vi "bbauv_acoustic_sbRIO_v2.vi"() -> ()   [LabVIEW 2012]
doc: "This VI will initialize the FPGA VI and read a user-defined number of samples from a DMA FIFO. When the data acquisition is complete this VI will read status information from the FPGA VI.\n\nFollow these instructions to run the VI.\n\n1. Select your RIO device from the dropdown.\n2. Set the sample period, number of samples to acquire per channel, and DMA block read size. \n\nNote: the block read size should be set to balance load on the host processor and the update rate of the user interface. A small block read size will update the user interface more often but will result in a higher load on the host processor."
uses:
  <vilib>/userdefined/High Color/nirio_resource_hc.ctl
  <vilib>/Analysis/3filter.llb/Butterworth Filter (DBL).vi
  <vilib>/FPGAPlugInAG/sbRIO-9612/niLvFpga_Open_sbRIO-9612.vi
  <vilib>/rvi/interface/common/dynamic/niFpgaDynamicAddResources.vi
  <vilib>/Utility/error.llb/Error Cluster From Error Code.vi
  <vilib>/FPGAPlugInAG/Dynamic/niLvFpga_Run_Dynamic.vi
  <vilib>/rvi/errors/niLvFpgaAdjustHostInterfaceError.vi
  <vilib>/RVI Host/nirviSupport.llb/nirviErrorClusterFromErrorCode.vi
  <vilib>/FPGAPlugInAG/Dynamic/niLvFpga_Close_Dynamic.vi
  <vilib>/rvi/interface/nirviOpenFPGA/nirviOpenFPGA.xnode
  FPGA Bitfiles/bbauvFPGA_FPGATarget2_NI9223User-Contr_AXBjtBmtN8Y.lvbitx
  NI 9223 User-Controlled IO Sampling (FPGA).vi
  <vilib>/rvi/interface/nirviMethod/nirviMethod.xnode
  <vilib>/rvi/interface/nirviReadWriteControl/nirviReadWriteControl.xnode
  <vilib>/rvi/interface/nirviCloseFPGA/nirviCloseFPGA.xnode
  <vilib>/rvi/errors/niLvFpgaMergeErrorWithErrorCode.vi
  <vilib>/rvi/interface/Simulation/niFpgaSimulationCallBeginRW.vi
  <vilib>/FPGAPlugInAG/Dynamic/niLvFpga_ReadFifo_Dynamic.vi
  <vilib>/rvi/interface/nirviMethod/StockFPGA_InlinedMethodWaitForSingleIRQ.vi
  <vilib>/FPGAPlugInAG/Dynamic/niLvFpga_WaitOnIrq_Dynamic.vi
  <vilib>/FPGAPlugInAG/Dynamic/niLvFpga_AcknowledgeIrq_Dynamic.vi
  NiFpgaLv.dll
  <vilib>/FPGAPlugInAG/Dynamic/niLvFpga_ConfigureFifo_Dynamic.vi
  <vilib>/FPGAPlugInAG/Dynamic/niLvFpga_StartFifo_Dynamic.vi
  <vilib>/Analysis/NI_AALBase.lvlib
  <vilib>/Analysis/NI_AALPro.lvlib
panel:
  in  "threshold ratio":dbl=3.0
  out "Sidemove":dbl
  out "Forward":dbl
  out "Threshold 3":dbl
  out "Threshold 2":dbl
  out "Threshold 1":dbl
  out "noise index":dbl[](array[numeric])
  out "Threshold 0":dbl
  out "Amplitude Spectrum":waveform(dbl)(graph)
  out "bad signal?":bool
  in  "Min Starting Index":i32=7000
  in  "Portion Duration":i32=1000
  out "amplitude 3":dbl
  out "amplitude 2":dbl
  out "amplitude 1":dbl
  out "amplitude 0":dbl
  in  "noise min":dbl=0.001
  out "Index 3":dbl
  out "Index 2":dbl
  out "Index 1":dbl
  out "Index 0":dbl
  out "current time":timestamp
  in  "Debug":bool=TRUE
  in  "Send to ROS":bool
  out "ROS  Error":bool
  out "dt1":dbl
  out "dt2":dbl
  out "dt3":dbl
  out "pitch":dbl
  out "yaw":dbl
  out "z":dbl
  out "y":dbl
  out "x":dbl
  in  "Mode":T1(ring)=enum."Use Far Field"
  in  "Altitude":dbl=2.0
  in  "Display Filtered Signal":bool=TRUE
  out "Ratio at Index (%)":dbl
  out "Selected Index":i32
  in  "Threshold":dbl=0.1
  in  "low cutoff freq: fl":dbl=20000.0
  in  "high cutoff freq: fh":dbl=30000.0
  out "Yaw Chart":dbl(graph)
  out "Ch0 Signal":dbl[](graph)
  out "#Elements Acquired":u32(graph)
  out "Extracted signal":dbl[][](graph)
  in  "Sampling Duration (us)":u32=2005000
  in  "RIO Device":T2="RIO0"
  out "Timed Out":bool
  out "Sample Gated":bool
  out "Overwrite":bool
  in  "Acquisition Stop":bool
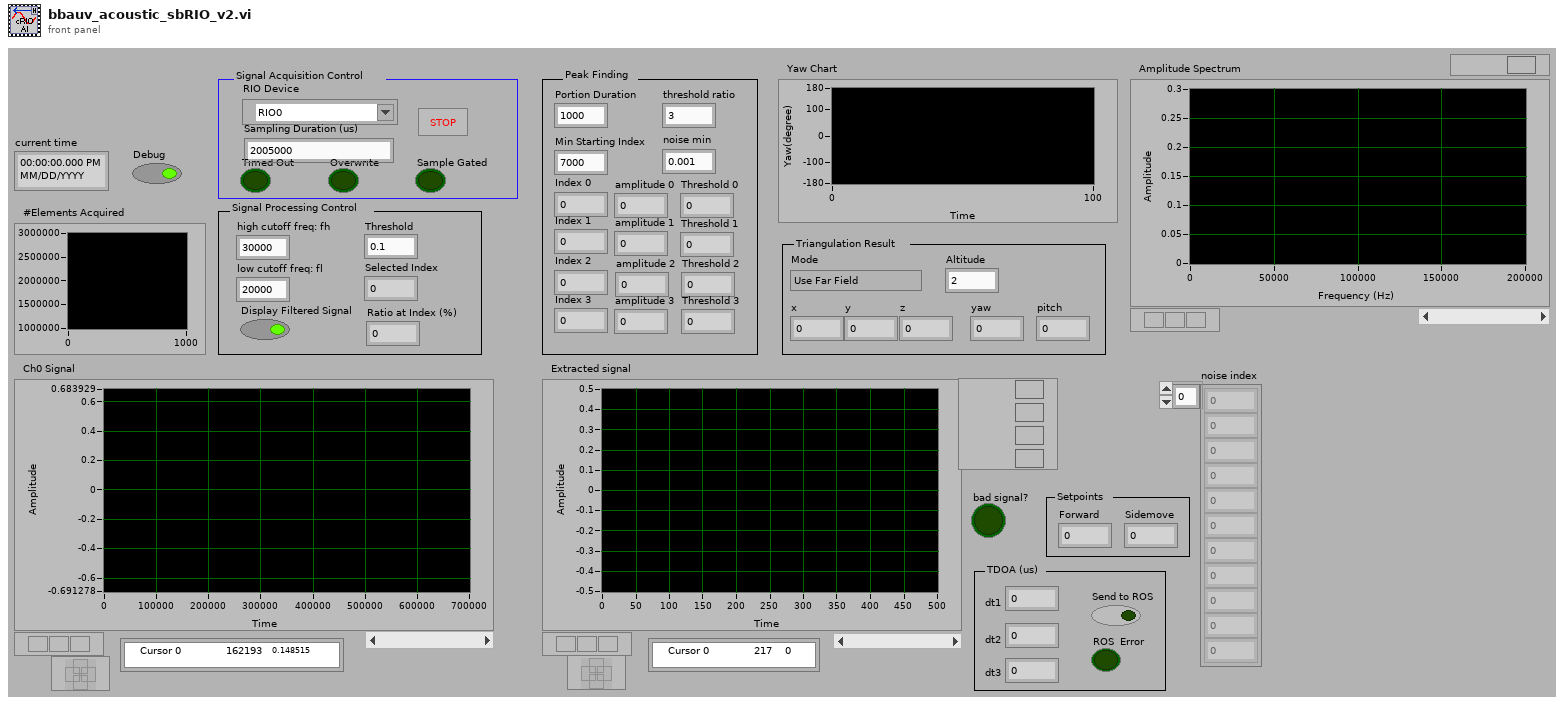
[diagram p1: front panel]
types:
  T1 = enum16{"Use Near Field", "Use Far Field", "Far Field with 3 hydrophones"}
  T2 = typedef "nirio_resource_hc.ctl" = tag
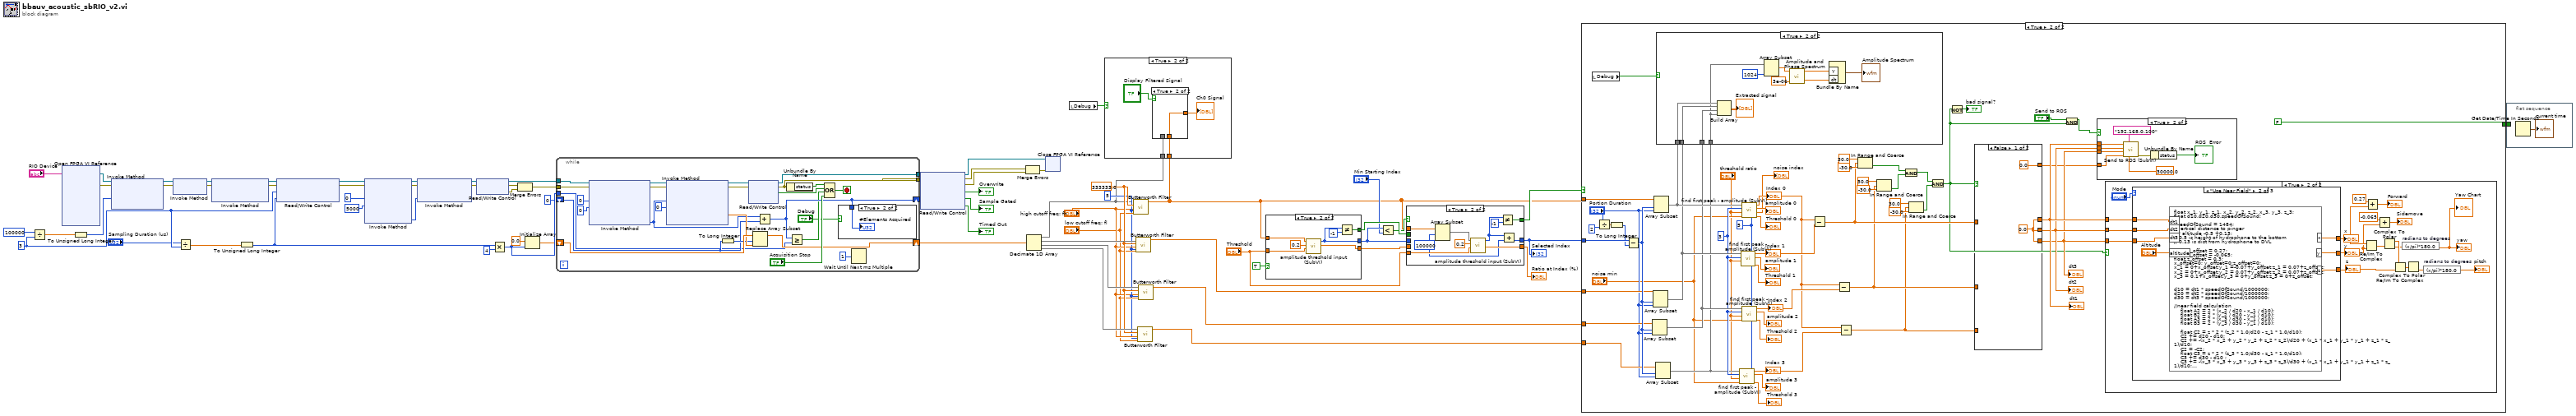
[diagram p0: block diagram]
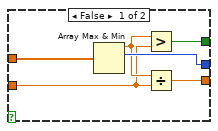
[diagram p5: hidden frame]
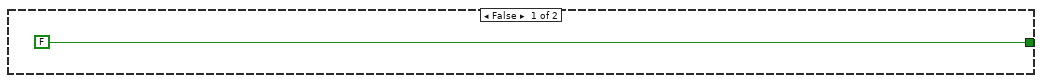
[diagram p6: hidden frame]
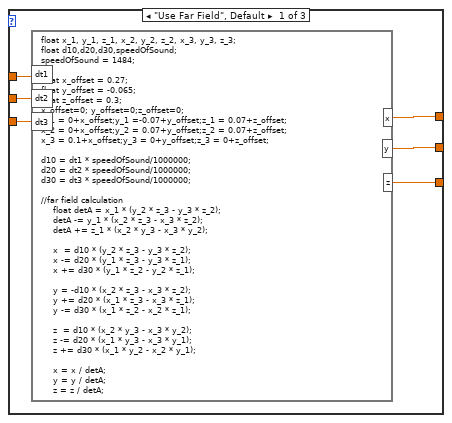
[diagram p8: hidden frame]
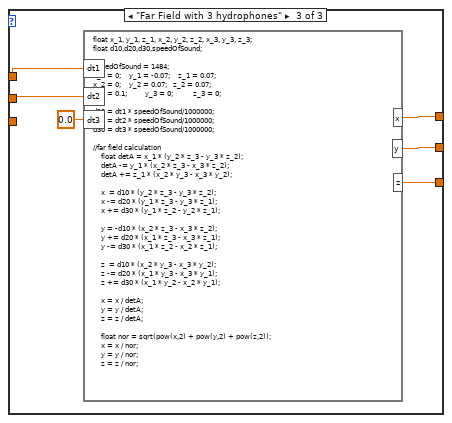
[diagram p9: hidden frame]
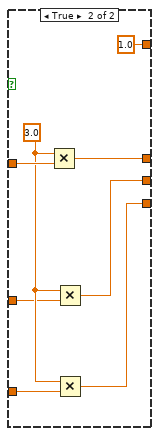
[diagram p11: hidden frame]
diagram:
  w6 = 5
  w12 = 333333.0
  w29 = u32 3
  n1 = Divide(x=u32 100000, y=w29) -> (x/y=w62:dbl)
  n2 = xnode "Open FPGA VI Reference"("resource name"="RIO Device") -> ("FPGA VI Reference Out"=w65:refnum<k20>, "error out"=w64:errorcluster)  [unwired: 1 in]
  n3 = To Unsigned Long Integer(number=w62) -> (unsigned 32bit integer=w63:u32)
  n4 = xnode "Invoke Method"("FPGA VI Reference In"=w65, "error in"=w64, "Requested Depth"=w63) -> ("FPGA VI Reference Out"=w67:refnum<k20>, "error out"=w66:errorcluster)  [unwired: 1 out]
  n5 = xnode "Invoke Method"("FPGA VI Reference In"=w67, "error in"=w66) -> ("FPGA VI Reference Out"=w56:refnum<k20>, "error out"=w55:errorcluster)
  n6 = Divide(x="Sampling Duration (us)", y=w29) -> (x/y=w27:dbl)
  n7 = xnode "Invoke Method"("FPGA VI Reference In"=w56, "error in"=w55) -> ("FPGA VI Reference Out"=w32:refnum<k20>, "error out"=w31:errorcluster)  [unwired: 1 in]
  n8 = To Unsigned Long Integer(number=w27) -> (unsigned 32bit integer=w25:u32)
  n9 = xnode "Read/Write Control"("FPGA VI Reference In"=w32, "error in"=w31, "Sample Period (uSec)"=w29, "Number of Samples"=w25) -> ("FPGA VI Reference Out"=w46:refnum<k20>, "error out"=w45:errorcluster)
  n10 = xnode "Invoke Method"("FPGA VI Reference In"=w46, "error in"=w45, "IRQ Number(s)"=0, "Timeout (ms)"=5000) -> ("FPGA VI Reference Out"=w43:refnum<k20>, "error out"=w44:errorcluster, "IRQ(s) Asserted"=w40:i32)  [unwired: 1 out]
  n11 = xnode "Invoke Method"("FPGA VI Reference In"=w43, "error in"=w44, "IRQ Number(s)"=w40) -> ("FPGA VI Reference Out"=w42:refnum<k20>, "error out"=w41:errorcluster)
  n12 = xnode "Read/Write Control"("FPGA VI Reference In"=w42, "error in"=w41) -> ("FPGA VI Reference Out"=w34:refnum<k20>, "error out"=w48:errorcluster, "Error Out"=w47:errorcluster)
  n13 = Multiply(x=w25, y=u32 4) -> (x*y=w59:u32)
  n14 = Merge Errors(w48, w47) -> (w33:errorcluster)
  n15 = Initialize Array(sgl 0.0, w59) -> (w35:sgl[])
  n16 = while {
    tunnel: w34 -> [w81]
    tunnel: w33 -> [w80]
    tunnel: [w89] -> w54
    tunnel: [w88] -> w53
    shift-right: [w71] -> _
    shift-left: u32 0 -> [w82]
    tunnel: w59 -> [w74]
    shift-right: [w84] -> w26
    shift-left: w35 -> [w90]
    stop <- w91 stop-if-true
    n17 = xnode "Invoke Method"("FPGA VI Reference In"=w81, "error in"=w80, "Number of Elements"=u32 0, "Timeout (ms)"=0) -> ("FPGA VI Reference Out"=w79:refnum<k20>, "error out"=w78:errorcluster, "Elements Remaining"=w72:u32)  [unwired: 1 out]
    n18 = xnode "Invoke Method"("FPGA VI Reference In"=w79, "error in"=w78, "Number of Elements"=w72, "Timeout (ms)"=0) -> ("FPGA VI Reference Out"=w94:refnum<k20>, "error out"=w93:errorcluster, "Data"=w85:sgl[])  [unwired: 1 out]
    n19 = To Long Integer(number=w82) -> (32bit integer=w83:i32)
    n20 = xnode "Read/Write Control"("FPGA VI Reference In"=w94, "error in"=w93) -> ("FPGA VI Reference Out"=w89:refnum<k20>, "error out"=w88:errorcluster, "Error"=w73:bool)  [unwired: 1 out]
    n21 = Replace Array Subset(array=w90, new element=w85, index=w83) -> (w84:sgl[])
    n22 = Add(x=w72, y=w82) -> (x+y=w71:u32)
    n23 = Unbundle By Name(w88) -> ("status"=w75:bool)
    n24 = Greater Or Equal?(x=w71, y=w74) -> (x >= y?=w70:bool)
    n25 = Compound Arithmetic op=OR(w75, w73, w70, "Acquisition Stop") -> (w91:bool)
    n26 = case shown="True" "Debug" {
      tunnel: w71 -> [_ w95]
      frame False {
      }
      frame True {
        "#Elements Acquired" <- w95
      }
    }
    n27 = Wait Until Next ms Multiple(millisecond multiple=u32 1) -> ()  [unwired: 1 out]
  }
  n28 = xnode "Read/Write Control"("FPGA VI Reference In"=w54, "error in"=w53) -> ("FPGA VI Reference Out"=w58:refnum<k20>, "error out"=w49:errorcluster, "Error Out"=w50:errorcluster, "Overwrite"=→"Overwrite":bool, "Sample Gated"=→"Sample Gated":bool, "Timed Out"=→"Timed Out":bool)
  n29 = Merge Errors(w49, w50) -> (w57:errorcluster)
  n30 = Decimate 1D Array(w26) -> (w4:sgl[], w15:sgl[], w14:sgl[], w13:sgl[])
  n31 = xnode "Close FPGA VI Reference"("FPGA VI Reference In"=w58, "error in"=w57) -> ()  [unwired: 1 out]
  n32 = local read "Debug"() -> (w3:bool)
  n33 = call-poly <vilib>:"Butterworth Filter.vi"("order"=w6, "low cutoff freq: fl"="low cutoff freq: fl", "high cutoff freq: fh"="high cutoff freq: fh", "sampling freq: fs"=w12, "X"=w4) -> ("Filtered X"=w1:dbl[])  [unwired: 3 in, 1 out]
  n34 = case shown="True" w3 {
    tunnel: w1 -> [_ w97]
    tunnel: w4 -> [_ w96]
    frame False {
    }
    frame True {
      n35 = case shown="True" "Display Filtered Signal" {
        tunnel: w96 -> [w100 _]
        tunnel: [w100 w101] -> w98
        tunnel: w97 -> [_ w101]
        frame False {
        }
        frame True {
        }
      }
      "Ch0 Signal" <- w98
    }
  }
  n36 = call-poly <vilib>:"Butterworth Filter.vi"("order"=w6, "low cutoff freq: fl"="low cutoff freq: fl", "high cutoff freq: fh"="high cutoff freq: fh", "sampling freq: fs"=w12, "X"=w15) -> ("Filtered X"=w9:dbl[])  [unwired: 3 in, 1 out]
  n37 = call-poly <vilib>:"Butterworth Filter.vi"("order"=w6, "low cutoff freq: fl"="low cutoff freq: fl", "high cutoff freq: fh"="high cutoff freq: fh", "sampling freq: fs"=w12, "X"=w13) -> ("Filtered X"=w7:dbl[])  [unwired: 3 in, 1 out]
  n38 = call-poly <vilib>:"Butterworth Filter.vi"("order"=w6, "low cutoff freq: fl"="low cutoff freq: fl", "high cutoff freq: fh"="high cutoff freq: fh", "sampling freq: fs"=w12, "X"=w14) -> ("Filtered X"=w8:dbl[])  [unwired: 3 in, 1 out]
  n39 = case shown="True" TRUE {
    tunnel: w1 -> [w107 w114]
    tunnel: [w104 w111] -> w21
    tunnel: [w105 w110] -> w18
    tunnel: [w106 w109] -> w23
    tunnel: "Threshold" -> [w102 w108]
    frame False {
      n40 = Array Max & Min(array=w107) -> (max value=w103:dbl, max index (indices)=w105:i32)  [unwired: 2 out]
      n41 = Greater?(x=w103, y=w102) -> (0:w106:bool)
      n42 = Divide(x=w103, y=w102) -> (x/y=w104:dbl)
    }
    frame True {
      n43 = call "amplitude threshold input (SubVI).vi"("threshold"=w108, "%max amplitude"=0.2, "Array"=w114) -> ("actual ratio (%)"=w111:dbl, "Index"=w110:i32)  [unwired: 7 in]
      n44 = Not Equal?(x=w110, y=-1) -> (x != y?=w109:bool)
    }
  }
  n45 = Less?(x=w18, y="Min Starting Index") -> (x < y?=w22:bool)
  n46 = case shown="True" w22 {
    tunnel: w23 -> [w117 _]
    tunnel: w21 -> [w115 _]
    tunnel: w1 -> [_ w127]
    tunnel: "Threshold" -> [_ w123]
    tunnel: [w117 w122] -> w16
    tunnel: [w116 w120] -> w17
    tunnel: [w115 w121] -> w19
    tunnel: w18 -> [w116 _]
    frame False {
    }
    frame True {
      w118 = 100000
      n47 = Array Subset(array=w127, index=w118) -> (w124:dbl[])  [unwired: 1 in]
      n48 = call "amplitude threshold input (SubVI).vi"("threshold"=w123, "%max amplitude"=0.2, "Array"=w124) -> ("actual ratio (%)"=w121:dbl, "Index"=w119:i32)  [unwired: 7 in]
      n49 = Not Equal?(x=w119, y=-1) -> (x != y?=w122:bool)
      n50 = Add(x=w119, y=w118) -> (x+y=w120:i32)
    }
  }
  "Ratio at Index (%)" <- w19
  "Selected Index" <- w17
  n51 = case shown="True" w16 {
    tunnel: w9 -> [_ w181]
    tunnel: w8 -> [_ w180]
    tunnel: w7 -> [_ w179]
    tunnel: w1 -> [_ w178]
    tunnel: w17 -> [_ w177]
    tunnel: [FALSE FALSE] -> w2
    frame False {
    }
    frame True {
      w129 = 5
      w142 = 3
      n52 = local read "Debug"() -> (w172:bool)
      n53 = Divide(x="Portion Duration", y=2) -> (x/y=w174:dbl)
      n54 = To Long Integer(number=w174) -> (32bit integer=w173:i32)
      n55 = Subtract(x=w177, y=w173) -> (x-y=w182:i32)
      n56 = Array Subset(array=w180, index=w182, length="Portion Duration") -> (w143:dbl[])
      n57 = Array Subset(array=w181, index=w182, length="Portion Duration") -> (w147:dbl[])
      n58 = Array Subset(array=w178, index=w182, length="Portion Duration") -> (w149:dbl[])
      n59 = Array Subset(array=w179, index=w182, length="Portion Duration") -> (w141:dbl[])
      n60 = case shown="True" w172 {
        tunnel: w147 -> [_ w248]
        tunnel: w143 -> [_ w247]
        tunnel: w141 -> [_ w238]
        tunnel: w149 -> [_ w246]
        frame False {
        }
        frame True {
          n61 = Build Array(w246, w248, w247, w238) -> (→"Extracted signal":dbl[][])
          n62 = Array Subset(array=w238, length=1024) -> (w242:dbl[])  [unwired: 1 in]
          n63 = call <vilib>:"Amplitude and Phase Spectrum.vi"("dt"=3e-06, "Signal (V)"=w242) -> ("df"=w239:dbl, "Amp Spectrum Mag (Vrms)"=w240:dbl[])  [unwired: 1 in, 1 out]
          n64 = Bundle By Name("Y"=w240, "dt"=w239) -> (→"Amplitude Spectrum":waveform(dbl))  [unwired: 1 in]
        }
      }
      n65 = call "find first peak - amplitude (SubVI).vi"("Noise length"=w129, "Noise min"="noise min", "threshold ratio"="threshold ratio", "width"=w142, "Array"=w141) -> ("Peak threshold"=→"Threshold 3":dbl, "peak amplitude"=→"amplitude 3":dbl, "Index"=w140:dbl)  [unwired: 2 in, 2 out]
      "Index 3" <- w140
      n66 = call "find first peak - amplitude (SubVI).vi"("Noise length"=w129, "threshold ratio"="threshold ratio", "width"=w142, "Array"=w147) -> ("Peak threshold"=→"Threshold 1":dbl, "peak amplitude"=→"amplitude 1":dbl, "Index"=w146:dbl)  [unwired: 3 in, 2 out]
      "Index 1" <- w146
      n67 = call "find first peak - amplitude (SubVI).vi"("Noise length"=w129, "Noise min"="noise min", "threshold ratio"="threshold ratio", "width"=w142, "Array"=w149) -> ("Peak threshold"=→"Threshold 0":dbl, "noise index"=→"noise index":dbl[], "peak amplitude"=→"amplitude 0":dbl, "Index"=w136:dbl)  [unwired: 2 in, 1 out]
      "Index 0" <- w136
      n68 = call "find first peak - amplitude (SubVI).vi"("Noise length"=w129, "Noise min"="noise min", "threshold ratio"="threshold ratio", "width"=w142, "Array"=w143) -> ("Peak threshold"=→"Threshold 2":dbl, "peak amplitude"=→"amplitude 2":dbl, "Index"=w144:dbl)  [unwired: 2 in, 2 out]
      "Index 2" <- w144
      n69 = Subtract(x=w136, y=w146) -> (x-y=w168:dbl)
      n70 = Subtract(x=w136, y=w144) -> (x-y=w165:dbl)
      n71 = Subtract(x=w136, y=w140) -> (x-y=w162:dbl)
      n72 = In Range and Coerce(upper limit=30.0, x=w168, lower limit=-30.0) -> (In Range?=w161:bool)  [unwired: 1 out]
      n73 = In Range and Coerce(upper limit=30.0, x=w165, lower limit=-30.0) -> (In Range?=w160:bool)  [unwired: 1 out]
      n74 = And(x=w161, y=w160) -> (x .and. y?=w159:bool)
      n75 = In Range and Coerce(upper limit=30.0, x=w162, lower limit=-30.0) -> (In Range?=w158:bool)  [unwired: 1 out]
      n76 = And(x=w159, y=w158) -> (x .and. y?=w150:bool)
      n77 = Not(x=w150) -> (.not. x?=→"bad signal?":bool)
      n78 = case shown="False" w150 {
        tunnel: w168 -> [_ w237]
        tunnel: w165 -> [_ w235]
        tunnel: w162 -> [_ w234]
        tunnel: [w228 w233] -> w155
        tunnel: [w228 w232] -> w154
        tunnel: [w228 w231] -> w153
        tunnel: [0.0 1.0] -> w152
        frame False {
          w228 = 0.0
        }
        frame True {
          w236 = 3.0
          n79 = Multiply(x=w236, y=w237) -> (x*y=w233:dbl)
          n80 = Multiply(x=w236, y=w235) -> (x*y=w232:dbl)
          n81 = Multiply(x=w236, y=w234) -> (x*y=w231:dbl)
        }
      }
      "dt1" <- w155
      "dt2" <- w154
      "dt3" <- w153
      n82 = And(x="Send to ROS", y=w150) -> (x .and. y?=w151:bool)
      n83 = case shown="True" w151 {
        tunnel: w155 -> [_ w223]
        tunnel: w154 -> [_ w222]
        tunnel: w153 -> [_ w221]
        tunnel: w152 -> [_ w220]
        frame False {
        }
        frame True {
          n84 = call "Send to ROS (SubVI).vi"("frequency"=30000.0, "ROS IP"="192.168.0.100", "Good signal?"=w220, "dt 3"=w221, "dt2"=w222, "dt 1"=w223) -> ("error out"=w226:errorcluster)  [unwired: 5 in]
          n85 = Unbundle By Name(w226) -> ("status"=→"ROS  Error":bool)
        }
      }
      n86 = case shown="True" w150 {
        tunnel: w155 -> [_ w191]
        tunnel: w154 -> [_ w190]
        tunnel: w153 -> [_ w189]
        frame False {
        }
        frame True {
          n87 = case shown="\"Use Near Field\"" "Mode" {
            tunnel: [w206 w213 w218] -> w188
            tunnel: [w205 w212 w217] -> w185
            tunnel: [w204 w211 w216] -> w195
            tunnel: w191 -> [w203 w209 w215]
            tunnel: w190 -> [w202 w208 w214]
            tunnel: w189 -> [w201 w207 _]
            frame "Use Far Field", Default {
              n88 = formula code="float x_1, y_1, z_1, x_2, y_2, z_2, x_3, y_3, z_3;\nfloat d10,d20,d30,speedOfSound;\nspeedOfSound = 1484;\n\nfloat x_offset = 0.27;\nfloat y_offset = -0.065;\nfloat z_offset = 0.3;\nx_offset=0; y_offset=0;z_offset=0;\nx_1 = 0+x_offset;y_1 =-0.07+y_offset;z_1 = 0.07+z_offset;\nx_2 = 0+x_offset;y_2 = 0.07+y_offset;z_2 = 0.07+z_offset;\nx_3 = 0.1+x_offset;y_3 = 0+y_offset;z_3 = 0+z_offset;\n\nd10 = dt1 * speedOfSound/1000000;\nd20 = dt2 * speedOfSound/1000000;\nd30 = dt3 * speedOfSound/1000000;\n\n//far field calculation\n    float detA = x_1 * (y_2 * z_3 - y_3 * z_2);\n    detA -= y_1 * (x_2 * z_3 - x_3 * z_2);\n    detA += z_1 * (x_2 * y_3 - x_3 * y_2);\n\n    x  = d10 * (y_2 * z_3 - y_3 * z_2);\n    x -= d20 * (y_1 * z_3 - y_3 * z_1);\n    x += d30 * (y_1 * z_2 - y_2 * z_1);\n\n    y = -d10 * (x_2 * z_3 - x_3 * z_2);\n    y += d20 * (x_1 * z_3 - x_3 * z_1);\n    y -= d30 * (x_1 * z_2 - x_2 * z_1);\n\n    z  = d10 * (x_2 * y_3 - x_3 * y_2);\n    z -= d20 * (x_1 * y_3 - x_3 * y_1);\n    z += d30 * (x_1 * y_2 - x_2 * y_1);\n\n    x = x / detA;\n    y = y / detA;\n    z = z / detA;\n\n    float nor = sqrt(pow(x,2) + pow(y,2) + pow(z,2));\n    x = x / nor;\n    y = y / nor;\n    z = z / nor;"("dt1"=w203, "dt2"=w202, "dt3"=w201) -> ("x"=w206:dbl, "y"=w205:dbl, "z"=w204:dbl)
            }
            frame "Use Near Field" {
              n89 = formula code="float x_1, y_1, z_1, x_2, y_2, z_2, x_3, y_3, z_3;\nfloat d10,d20,d30,speedOfSound;\n\nspeedOfSound = 1484;\n//vertical distance to pinger\nz= altitude -0.5 +0.13;\n// 0.5 is height of hydrophone to the bottom\n// 0.13 is dist from hydrophone to DVL\n\nfloat x_offset = 0.27;\nfloat y_offset = -0.065;\nfloat z_offset = 0.3;\nx_offset=0; y_offset=0;z_offset=0;\nx_1 = 0+x_offset;y_1 =-0.07+y_offset;z_1 = 0.07+z_offset;\nx_2 = 0+x_offset;y_2 = 0.07+y_offset;z_2 = 0.07+z_offset;\nx_3 = 0.1+x_offset;y_3 = 0+y_offset;z_3 = 0+z_offset;\n\n\nd10 = dt1 * speedOfSound/1000000;\nd20 = dt2 * speedOfSound/1000000;\nd30 = dt3 * speedOfSound/1000000;\n\n//near field calculation\n    float A2 = 2 * (x_2 / d20 - x_1 / d10);\n    float B2 = 2 * (y_2 / d20 - y_1 / d10);\n    float A3 = 2 * (x_3 / d30 - x_1 / d10);\n    float B3 = 2 * (y_3 / d30 - y_1 / d10);\n    \n    float C2 = z * 2 * (z_2 * 1.0/d20 - z_1 * 1.0/d10);\n    C2 += d20 - d10;\n    C2 += -(x_2 * x_2 + y_2 * y_2 + z_2 * z_2)/d20 + (x_1 * x_1 + y_1 * y_1 + z_1 * z_1)/d10;\n    C2 = -C2;\n    float C3 = z * 2 * (z_3 * 1.0/d30 - z_1 * 1.0/d10);\n    C3 += d30 - d10 ;\n    C3 += -(x_3 * x_3 + y_3 * y_3 + z_3 * z_3)/d30 + (x_1 * x_1 + y_1 * y_1 + z_1 * z_1)/d10;\n    C3 = -C3;\n\n    if (A2*B3 == A3*B2) {\n        x = 0;\n        y = 0;\n    }\n    else {\n        x = (C2 * B3 - C3 * B2) / (A2 * B3 - A3 * B2);\n        y = (C3 * A2 - C2 * A3) / (B3 * A2 - B2 * A3);\n    }"("dt1"=w209, "dt2"=w208, "dt3"=w207, "altitude"="Altitude") -> ("x"=w213:dbl, "y"=w212:dbl, "z"=w211:dbl)
            }
            frame "Far Field with 3 hydrophones" {
              n90 = formula code="float x_1, y_1, z_1, x_2, y_2, z_2, x_3, y_3, z_3;\nfloat d10,d20,d30,speedOfSound;\n\nspeedOfSound = 1484;\nx_1 = 0;    y_1 = -0.07;    z_1 = 0.07;\nx_2 = 0;    y_2 = 0.07;   z_2 = 0.07;\nx_3 = 0.1;         y_3 = 0;          z_3 = 0;\n\nd10 = dt1 * speedOfSound/1000000;\nd20 = dt2 * speedOfSound/1000000;\nd30 = dt3 * speedOfSound/1000000;\n\n//far field calculation\n    float detA = x_1 * (y_2 * z_3 - y_3 * z_2);\n    detA -= y_1 * (x_2 * z_3 - x_3 * z_2);\n    detA += z_1 * (x_2 * y_3 - x_3 * y_2);\n\n    x  = d10 * (y_2 * z_3 - y_3 * z_2);\n    x -= d20 * (y_1 * z_3 - y_3 * z_1);\n    x += d30 * (y_1 * z_2 - y_2 * z_1);\n\n    y = -d10 * (x_2 * z_3 - x_3 * z_2);\n    y += d20 * (x_1 * z_3 - x_3 * z_1);\n    y -= d30 * (x_1 * z_2 - x_2 * z_1);\n\n    z  = d10 * (x_2 * y_3 - x_3 * y_2);\n    z -= d20 * (x_1 * y_3 - x_3 * y_1);\n    z += d30 * (x_1 * y_2 - x_2 * y_1);\n\n    x = x / detA;\n    y = y / detA;\n    z = z / detA;\n\n    float nor = sqrt(pow(x,2) + pow(y,2) + pow(z,2));\n    x = x / nor;\n    y = y / nor;\n    z = z / nor;"("dt1"=w215, "dt2"=w214, "dt3"=0.0) -> ("x"=w218:dbl, "y"=w217:dbl, "z"=w216:dbl)
            }
          }
          "x" <- w188
          "y" <- w185
          "z" <- w195
          n91 = Re/Im To Complex(1:w185, 2:w188) -> (0:w193:cdb)
          n92 = Add(x=0.27, y=w188) -> (x+y=→"Forward":dbl)
          n93 = Add(x=-0.065, y=w185) -> (x+y=→"Sidemove":dbl)
          n94 = Complex To Polar(r * e^(i*theta)=w193) -> (r=w196:dbl, theta=w194:dbl)
          n95 = Re/Im To Complex(1:w195, 2:w196) -> (0:w197:cdb)
          n96 = expression code="(x/pi)*180.0"(w194) -> (→"yaw" →"Yaw Chart":dbl)
          n97 = Complex To Polar(r * e^(i*theta)=w197) -> (theta=w199:dbl)  [unwired: 1 out]
          n98 = expression code="(x/pi)*180.0"(w199) -> (→"pitch":dbl)
        }
      }
    }
  }
  n99 = flat-sequence {
    tunnel: w2 -> [_]
    frame #0 {
      n100 = Get Date/Time In Seconds() -> (seconds since 1Jan1904=→"current time":timestamp)
    }
  }
